vi "Waveform Trigger and Trim.vi"(11 "Waveforms In":waveform(dbl)[](array[waveform])=[{"t0"=timestamp(3462637932.578125 s since 1904-01-01), "dt"=5.8800000000000005e-06, "Y"=array[5000 elements]}, {"t0"=timestamp(3462637932.578125 s since 1904-01-01), "dt"=5.8800000000000005e-06, "Y"=array[5000 elements]}]) -> (3 "Waveforms Out":waveform(dbl)[](array[waveform]))   [LabVIEW 2010]
uses:
  <vilib>/measure/mamon.llb/Trigger Detection for 1 Channel.vi
  <vilib>/measure/NI_MAPro.lvlib
panel:
  out "Input Waveforms":waveform(dbl)[](graph)
  out "First Waveform":waveform(dbl)[](graph)
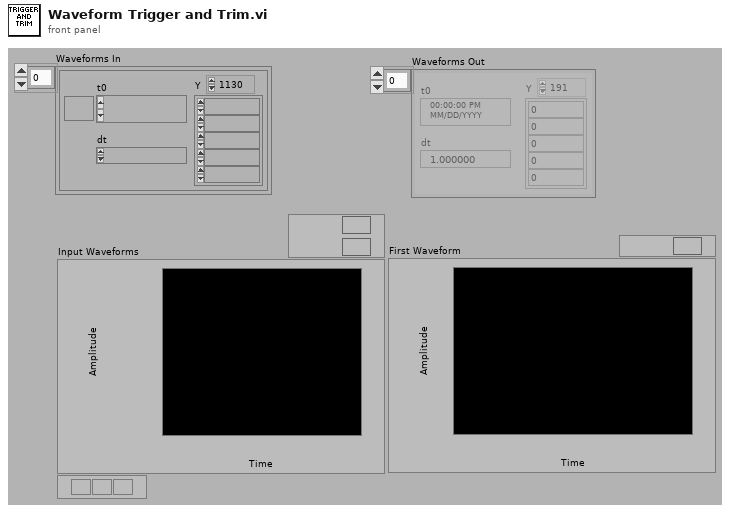
[diagram p1: front panel]
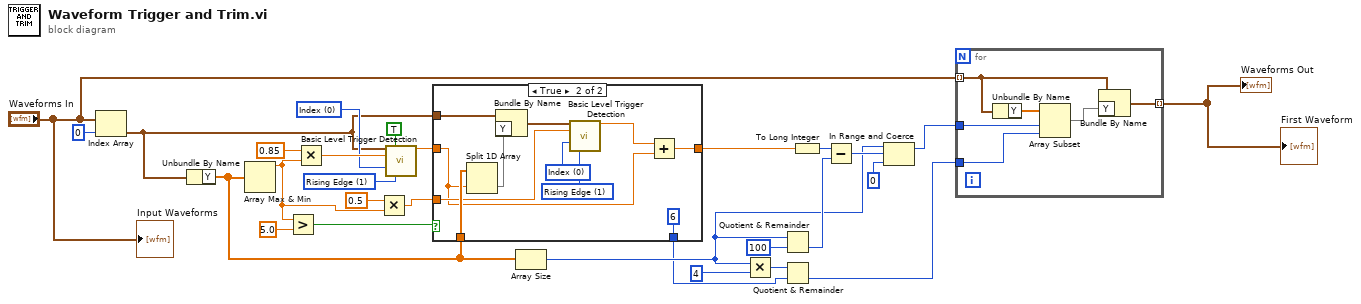
[diagram p0: block diagram]
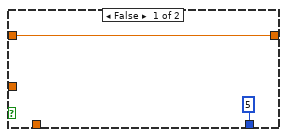
[diagram p2: hidden frame]
diagram:
  w24 = u16 1 items=["Falling Edge", "Rising Edge"] ("trigger slope")
  w25 = u16 0 items=["Index", "Time"] ("location mode")
  n1 = Index Array(array="Waveforms In", index=0) -> (element=w8:waveform(dbl))
  n2 = Unbundle By Name(w8) -> ("Y"=w7:dbl[])
  n3 = Array Max & Min(array=w7) -> (max value=w5:dbl)  [unwired: 3 out]
  n4 = Greater?(x=w5, y=5.0) -> (0:w12:bool)
  n5 = Multiply(x=0.85, y=w5) -> (x*y=w26:dbl)
  n6 = Multiply(x=0.5, y=w5) -> (x*y=w4:dbl)
  n7 = call-poly <vilib>:"Basic Level Trigger Detection.vi"("signal in"=w8, "reset"=TRUE, "level"=w26, "location mode"=w25, "trigger slope"=w24) -> ("trigger location"=w10:dbl)  [unwired: 8 in, 2 out]
  n8 = case shown="True" w12 {
    tunnel: [5 ("y") 6 ("y")] -> w11
    tunnel: w10 -> [w29 w33]
    tunnel: [w29 w31] -> w9
    tunnel: w8 -> [_ w40]
    tunnel: w7 -> [_ w39]
    tunnel: w4 -> [_ w34]
    frame False {
    }
    frame True {
      w35 = u16 1 items=["Falling Edge", "Rising Edge"] ("trigger slope")
      w36 = u16 0 items=["Index", "Time"] ("location mode")
      n9 = Split 1D Array(array=w39, index=w33) -> (second subarray=w38:dbl[])  [unwired: 1 out]
      n10 = Bundle By Name(cluster=w40, "Y"=w38) -> (w37:waveform(dbl))
      n11 = call-poly <vilib>:"Basic Level Trigger Detection.vi"("signal in"=w37, "level"=w34, "location mode"=w36, "trigger slope"=w35) -> ("trigger location"=w32:dbl)  [unwired: 9 in, 2 out]
      n12 = Add(x=w32, y=w33) -> (x+y=w31:dbl)
    }
  }
  n13 = Array Size(array=w7) -> (size(s)=w16:i32)
  n14 = Multiply(x=w16, y=4) -> (x*y=w22:i32)
  n15 = Quotient & Remainder(x=w16, y=100) -> (floor(x/y)=w18:i32)  [unwired: 1 out]
  n16 = Quotient & Remainder(x=w22, y=w11) -> (floor(x/y)=w21:i32)  [unwired: 1 out]
  n17 = To Long Integer(number=w9) -> (32bit integer=w19:i32)
  n18 = Subtract(x=w19, y=w18) -> (x-y=w17:i32)
  n19 = In Range and Coerce(upper limit=w16, x=w17, lower limit=0) -> (coerced(x)=w14:i32)  [unwired: 1 out]
  n20 = for {
    tunnel: "Waveforms In" -> [w44] mode=indexing
    tunnel: w21 -> [w46]
    tunnel: w14 -> [w45]
    tunnel: [w42] -> w1 mode=indexing
    n21 = Unbundle By Name(w44) -> ("Y"=w47:dbl[])
    n22 = Array Subset(array=w47, index=w45, length=w46) -> (w43:dbl[])
    n23 = Bundle By Name(cluster=w44, "Y"=w43) -> (w42:waveform(dbl))
  }
  "Waveforms Out" <- w1
  "First Waveform" <- w1
  "Input Waveforms" <- "Waveforms In"
